vi "System-CAN-Interface.vi"() -> ()   [LabVIEW 2016, in "DSI-RT.lvlib"]
uses:
  DSI-RT.lvlib
  <vilib>/RioEmbeddedCAN/RioEmbeddedCAN.llb/CANFrameControl.ctl
  <vilib>/addons/Software Calibration Management/xSCM/SubVIs/Variant Type Index.vi
  <vilib>/addons/Software Calibration Management/xSCM/SubVIs/Variant Element By Index.vi
  <vilib>/addons/Software Calibration Management/xSCM/SubVIs/Variant Element Set.vi
  <vilib>/addons/Software Calibration Management/xSCM/Get/Get Variant.vi
  <vilib>/addons/Software Calibration Management/xSCM/SubVIs/Variant Data Index.vi
  <vilib>/addons/Software Calibration Management/xSCM/Set/Set Variant.vi
  <vilib>/addons/Software Calibration Management/xSCM/CalPoint.xnode
  <vilib>/addons/Software Calibration Management/xSCM/ni_scm.dll
  <vilib>/addons/Software Calibration Management/xSCM/SCM-API.lvlib
panel:
  out "Period [ms]":u32
  out "Reset":bool
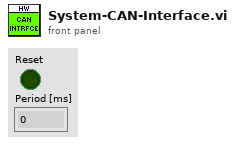
[diagram p1: front panel]
types:
  T1 = cluster{"_Name":string, "_Units":string, "_Identifier":u32, "_Disable":bool, "_Type":u16, "_Scaling Factor":sgl, "_Offset":sgl, "_ExtID":bool, "_Min":sgl, "_Max":sgl, "_Number of Bits":u8, "_Start Bit":u8, "_Byte Order":u8, "ID in":cluster{"ID":u32, "Element":i32[]}}[]
  T2 = cluster{"StartBit":u8, "Num Bits":u8, "Byte Order":u8, "Data Type":u8}
  T3 = cluster{"ScalingFactor":sgl, "Offset":sgl, "Maximum":sgl, "Minimum":sgl}
  T4 = typedef "CANFrameControl.ctl" = cluster{"identifier":u32, "extended?":bool, "type":u8, "payload":u8[]}
  T5 = cluster{"_Name":string, "_Units":string, "_Identifier":u32, "_Disable":bool, "_Type":u16, "_Scaling Factor":sgl, "_Offset":sgl, "_ExtID":bool, "_Min":sgl, "_Max":sgl, "_Number of Bits":u8, "_Start Bit":u8, "_Byte Order":u8, "ID in":cluster{"ID":u32, "Element":i32[]}}
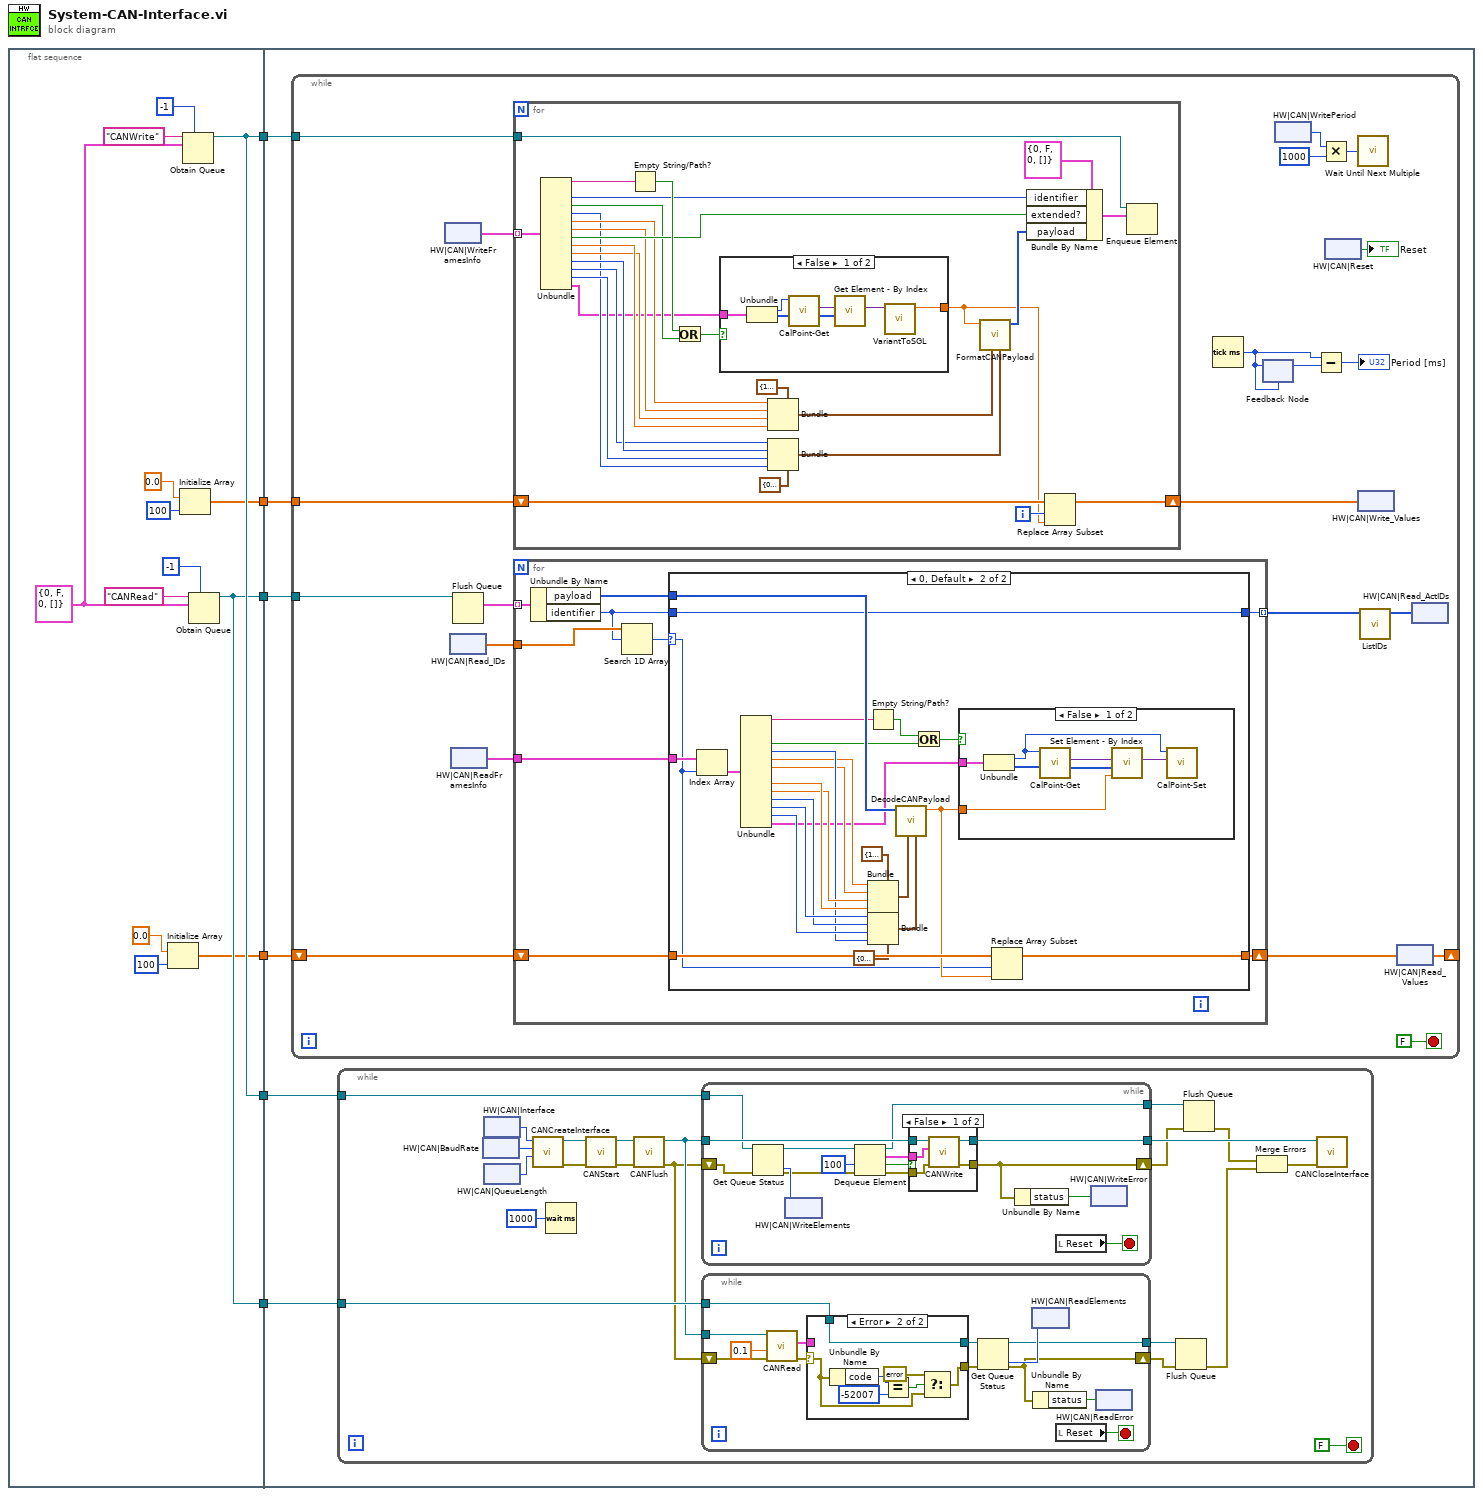
[diagram p0: block diagram]
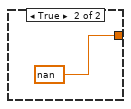
[diagram p4: hidden frame]
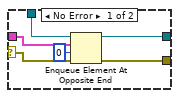
[diagram p5: hidden frame]
diagram:
  n1 = flat-sequence {
    tunnel: [w16] -> w6
    tunnel: [w15] -> w5
    tunnel: [w16] -> w4
    tunnel: [w15] -> w3
    tunnel: [w12] -> w2
    tunnel: [w7] -> w1
    tunnel: w6 -> [w25]
    tunnel: w5 -> [w24]
    tunnel: w4 -> [w23]
    tunnel: w3 -> [w20]
    tunnel: w2 -> [w22]
    tunnel: w1 -> [w21]
    frame #0 {
      w17 = T4 {"identifier"=0, "extended?"=FALSE, "type"=0, "payload"=[]} ("CAN frame")
      n2 = Initialize Array(sgl 0.0 ("Value"), 100 ("dimension size")) -> (w12:sgl[])
      n3 = Initialize Array(sgl 0.0 ("Value"), 100 ("dimension size")) -> (w7:sgl[])
      n4 = Obtain Queue(max queue size (-1, unlimited)=-1, name (unnamed)="CANWrite", element data type=w17) -> (queue out=w16:refnum<queue>)  [unwired: 2 in, 2 out]
      n5 = Obtain Queue(max queue size (-1, unlimited)=-1, name (unnamed)="CANRead", element data type=w17) -> (queue out=w15:refnum<queue>)  [unwired: 2 in, 2 out]
    }
    frame #1 {
      n6 = while {
        tunnel: w25 -> [w43]
        tunnel: w24 -> [w42]
        shift-right: [w38] -> _
        shift-left: w22 -> [w39]
        tunnel: w21 -> [w37]
        stop <- FALSE stop-if-true
        n7 = xnode "HW|CAN|WriteFramesInfo"() -> ("Value"=w26:T1)
        n8 = xnode "HW|CAN|Read_IDs"() -> ("Value"=w27:sgl[])
        n9 = xnode "HW|CAN|ReadFramesInfo"() -> ("Value"=w28:T1)
        n10 = Flush Queue(queue=w42) -> (remaining elements=w44:T4[])  [unwired: 1 in, 2 out]
        n11 = for {
          tunnel: w43 -> [w182]
          shift-right: [w178] -> w36
          shift-left: w37 -> [w181]
          tunnel: w26 -> [w171] mode=indexing
          i -> [w180]
          n12 = Unbundle(w171) -> ("_Name"=w167:string, "_Identifier"=w170:u32, "_Disable"=w168:bool, "_Type"=w159:u16, "_Scaling Factor"=w166:sgl, "_Offset"=w165:sgl, "_ExtID"=w169:bool, "_Min"=w164:sgl, "_Max"=w163:sgl, "_Number of Bits"=w162:u8, "_Start Bit"=w161:u8, "_Byte Order"=w160:u8, "ID in"=w158:cluster{"ID":u32, "Element":i32[]})  [unwired: 1 out]
          n13 = Empty String/Path?(string/path=w167) -> (empty?=w172:bool)
          n14 = Or(x=w172, y=w168) -> (x .or. y?=w173:bool)
          n15 = case shown="False" w173 {
            tunnel: [w186 sgl nan ("Value")] -> w179
            tunnel: w158 -> [w188 _]
            frame False {
              n16 = Unbundle(w188) -> ("ID"=w189:u32, "Element"=w191:i32[])
              n17 = call-poly <vilib>:"CalPoint-Get.vi"("ID"=w189) -> ("Data"=w190:variant)  [unwired: 10 in]
              n18 = call <vilib>:"Get Element - By Index.vi"("Elements"=w191, "Variant"=w190) -> ("Element"=w187:variant)  [unwired: 8 in, 1 out]
              n19 = call "VariantToSGL.vi"("Element"=w187) -> ("Numeric"=w186:sgl)  [unwired: 10 in]
            }
            frame True {
            }
          }
          n20 = Bundle(cluster=T3 {"ScalingFactor"=1.0, "Offset"=0.0, "Maximum"=1.0, "Minimum"=0.0} ("DataFormat"), "ScalingFactor"=w166, "Offset"=w165, "Maximum"=w163, "Minimum"=w164) -> (w174:T3)
          n21 = Bundle(cluster=T2 {"StartBit"=0, "Num Bits"=0, "Byte Order"=1, "Data Type"=1} ("ByteFormat"), "StartBit"=w161, "Num Bits"=w162, "Byte Order"=w160, "Data Type"=w159) -> (w175:T2)
          n22 = call "FormatCANPayload.vi"("ByteFormat"=w175, "DataFormat"=w174, "Value"=w179) -> ("payload"=w184:u8[])  [unwired: 8 in]
          n23 = Bundle By Name(cluster=T4 {"identifier"=0, "extended?"=FALSE, "type"=0, "payload"=[]} ("CAN frame"), "identifier"=w170, "extended?"=w169, "payload"=w184) -> (w183:T4)
          n24 = Replace Array Subset(array=w181, new element=w179, index=w180) -> (w178:sgl[])
          n25 = Enqueue Element(queue=w182, element=w183) -> ()  [unwired: 2 in, 3 out]
        }
        n26 = for {
          tunnel: w27 -> [w122]
          tunnel: w28 -> [w124]
          tunnel: w44 -> [w123] mode=indexing
          tunnel: [w118] -> w41 mode=indexing
          shift-right: [w116] -> w38
          shift-left: w39 -> [w117]
          n27 = Unbundle By Name(w123) -> ("payload"=w120:u8[], "identifier"=w119:u32)
          n28 = Search 1D Array(1D array=w122, element=w119) -> (index of element=w121:i32)  [unwired: 1 in]
          n29 = case shown="0, Default" w121 {
            selector: w121 -> [_ w128]
            tunnel: w124 -> [_ w141]
            tunnel: w120 -> [_ w151]
            tunnel: w119 -> [w126 w150]
            tunnel: [w126 w150] -> w118
            tunnel: w117 -> [w125 w149]
            tunnel: [w125 w148] -> w116
            frame -1 {
            }
            frame 0, Default {
              n30 = Index Array(array=w141, index=w128) -> (element=w140:T5)
              n31 = Unbundle(w140) -> ("_Name"=w139:string, "_Disable"=w137:bool, "_Type"=w131:u16, "_Scaling Factor"=w130:sgl, "_Offset"=w129:sgl, "_Min"=w133:sgl, "_Max"=w132:sgl, "_Number of Bits"=w134:u8, "_Start Bit"=w135:u8, "_Byte Order"=w136:u8, "ID in"=w127:cluster{"ID":u32, "Element":i32[]})  [unwired: 3 out]
              n32 = Empty String/Path?(string/path=w139) -> (empty?=w138:bool)
              n33 = Bundle(cluster=T3 {"ScalingFactor"=1.0, "Offset"=0.0, "Maximum"=1.0, "Minimum"=0.0} ("DataFormat"), "ScalingFactor"=w130, "Offset"=w129, "Maximum"=w132, "Minimum"=w133) -> (w143:T3)
              n34 = Bundle(cluster=T2 {"StartBit"=0, "Num Bits"=0, "Byte Order"=1, "Data Type"=1} ("ByteFormat"), "StartBit"=w135, "Num Bits"=w134, "Byte Order"=w136, "Data Type"=w131) -> (w144:T2)
              n35 = call "DecodeCANPayload.vi"("ByteFormat"=w144, "DataFormat"=w143, "payload"=w151) -> ("Value"=w147:sgl)  [unwired: 8 in]
              n36 = Or(x=w138, y=w137) -> (x .or. y?=w142:bool)
              n37 = case shown="False" w142 {
                tunnel: w147 -> [w153 _]
                tunnel: w127 -> [w152 _]
                frame False {
                  n38 = Unbundle(w152) -> ("ID"=w157:u32, "Element"=w155:i32[])
                  n39 = call-poly <vilib>:"CalPoint-Get.vi"("ID"=w157) -> ("Data"=w154:variant)  [unwired: 10 in]
                  n40 = call <vilib>:"Set Element - By Index.vi"("Element"=w153, "Elements"=w155, "Variant"=w154) -> ("Variant"=w156:variant)  [unwired: 8 in]
                  n41 = call-poly <vilib>:"CalPoint-Set.vi"("Data"=w156, "ID"=w157) -> ()  [unwired: 10 in]
                }
                frame True {
                }
              }
              n42 = Replace Array Subset(array=w149, new element=w147, index=w128) -> (w148:sgl[])
            }
          }
        }
        n43 = Tick Count (ms)() -> (millisecond timer value=w29:u32)
        n44 = feedback-in #1(w29) -> ()
        n45 = feedback #1(w29) -> (w30:u32)
        n46 = xnode "HW|CAN|WritePeriod"() -> ("Value"=w35:u32)
        n47 = Subtract(x=w29, y=w30) -> (x-y=→"Period [ms]":u32)
        n48 = Multiply(x=w35, y=u32 1000) -> (x*y=w33:u32)
        n49 = xnode "HW|CAN|Reset"() -> ("Value"=→"Reset":bool)
        n50 = call "Wait Until Next Multiple"("Count(uSec)"=w33) -> ()  [unwired: 1 out]
        n51 = xnode "HW|CAN|Write_Values"("Value"=w36) -> ()
        n52 = call "ListIDs.vi"("New IDs"=w41) -> ("Buffer"=w40:u32[])  [unwired: 10 in]
        n53 = xnode "HW|CAN|Read_Values"("Value"=w38) -> ()
        n54 = xnode "HW|CAN|Read_ActIDs"("Value"=w40) -> ()
      }
      n55 = while {
        tunnel: w23 -> [w209]
        tunnel: w20 -> [w203]
        stop <- FALSE stop-if-true
        n56 = xnode "HW|CAN|BaudRate"() -> ("Value"=w212:u32)
        n57 = xnode "HW|CAN|Interface"() -> ("Value"=w213:u8)
        n58 = xnode "HW|CAN|QueueLength"() -> ("Value"=w211:u8)
        n59 = call <vilib>:"CANCreateInterface.vi"("receive queue size (5)"=w211, "baud rate (125000 bps)"=w212, "interface index"=w213) -> ("error out"=w207:errorcluster, "interface object out"=w206:refnum<k20>)  [unwired: 7 in]
        n60 = Wait (ms)(milliseconds to wait=u32 1000) -> ()  [unwired: 1 out]
        n61 = call <vilib>:"CANStart.vi"("error in (no error)"=w207, "interface object in"=w206) -> ("error out"=w204:errorcluster, "interface object out"=w205:refnum<k20>)  [unwired: 8 in]
        n62 = call <vilib>:"CANFlush.vi"("error in (no error)"=w204, "interface object in"=w205) -> ("error out"=w201:errorcluster, "interface object out"=w202:refnum<k20>)  [unwired: 8 in]
        n63 = while {
          tunnel: w202 -> [w280]
          shift-right: [w269] -> w195
          shift-left: w201 -> [w273]
          tunnel: w209 -> [w276]
          tunnel: [w270] -> w208
          tunnel: [w266] -> w198
          stop <- w267 stop-if-true
          n64 = Get Queue Status(queue=w276, error in (no error)=w273) -> (queue out=w277:refnum<queue>, error out=w271:errorcluster, # elements in queue=w275:i32)  [unwired: 1 in, 5 out]
          n65 = xnode "HW|CAN|WriteElements"("Value"=w275) -> ()
          n66 = Dequeue Element(queue=w277, timeout in ms (-1)=100, error in (no error)=w271) -> (queue out=w266:refnum<queue>, element=w279:T4, timed out?=w278:bool, error out=w274:errorcluster)
          n67 = case shown="False" w278 {
            tunnel: w280 -> [w293 w295]
            tunnel: w279 -> [w289 _]
            tunnel: w274 -> [w292 w294]
            tunnel: [w291 w295] -> w270
            tunnel: [w290 w294] -> w269
            frame False {
              n68 = call <vilib>:"CANWrite.vi"("error in (no error)"=w292, "CAN frame"=w289, "interface object in"=w293) -> ("error out"=w290:errorcluster, "interface object out"=w291:refnum<k20>)  [unwired: 7 in]
            }
            frame True {
            }
          }
          n69 = Unbundle By Name(w269) -> ("status"=w268:bool)
          n70 = local read "Reset"() -> (w267:bool)
          n71 = xnode "HW|CAN|WriteError"("Value"=w268) -> ()
        }
        n72 = while {
          tunnel: w203 -> [w238]
          tunnel: w202 -> [w237]
          shift-right: [w235] -> w196
          shift-left: w201 -> [w236]
          tunnel: [w232] -> w197
          stop <- w233 stop-if-true
          n73 = call <vilib>:"CANRead.vi"("error in (no error)"=w236, "timeout (0 s)"=0.1, "interface object in"=w237) -> ("error out"=w243:errorcluster, "CAN frame"=w240:T4)  [unwired: 5 in, 2 out]
          n74 = case shown="Error" w243 {
            selector: w243 -> [w255 w262]
            tunnel: w240 -> [w258 _]
            tunnel: [w256 w260] -> w241
            tunnel: [w254 w261] -> w244
            tunnel: w238 -> [w253 w260]
            frame No Error {
              n75 = Enqueue Element At Opposite End(queue=w253, element=w258, timeout in ms (-1)=0, error in (no error)=w255) -> (queue out=w256:refnum<queue>, error out=w254:errorcluster)  [unwired: 1 out]
            }
            frame Error {
              n76 = Unbundle By Name(w262) -> ("code"=w265:i32)
              n77 = Equal?(x=w265, y=-52007) -> (x = y?=w263:bool)
              n78 = Select(t=errorcluster {"status"=FALSE, "code"=0, "source"=""}, s=w263, f=w262) -> (s? t:f=w261:errorcluster)
            }
          }
          n79 = Get Queue Status(queue=w241, error in (no error)=w244) -> (queue out=w232:refnum<queue>, error out=w235:errorcluster, # elements in queue=w242:i32)  [unwired: 1 in, 5 out]
          n80 = xnode "HW|CAN|ReadElements"("Value"=w242) -> ()
          n81 = Unbundle By Name(w235) -> ("status"=w234:bool)
          n82 = local read "Reset"() -> (w233:bool)
          n83 = xnode "HW|CAN|ReadError"("Value"=w234) -> ()
        }
        n84 = Flush Queue(queue=w197, error in (no error)=w196) -> (error out=w193:errorcluster)  [unwired: 2 out]
        n85 = Flush Queue(queue=w198, error in (no error)=w195) -> (error out=w194:errorcluster)  [unwired: 2 out]
        n86 = Merge Errors(w194, w193) -> (w200:errorcluster)
        n87 = call <vilib>:"CANCloseInterface.vi"("error in (no error)"=w200, "interface object in"=w208) -> ()  [unwired: 9 in, 1 out]
      }
    }
  }
